vi "Convert to GRobot.vi"(8 "error in (no error)":errorcluster, 10 "scale":dbl=1.0, 11 "Robot In":refnum<class "NI_Robotics_Serial Robot Arm.lvclass">) -> (0 "error out":errorcluster, 2 "Robot Elements":T1[](array[typedef]), 3 "Robot Out":refnum<class "NI_Robotics_Serial Robot Arm.lvclass">)   [LabVIEW 2017, in "NI_Robotics_3DKinematics.lvlib"]
uses:
  <vilib>/robotics/Kinematics/Plotting/NI_Robotics_3DKinematics.lvlib
  <vilib>/robotics/Kinematics/Plotting/Tree Element.ctl
  <vilib>/robotics/Kinematics/Plotting/Element Type.ctl
  <vilib>/robotics/Kinematics/Plotting/Joint Type.ctl
  <vilib>/robotics/Kinematics/Robot/NI_Robotics_Serial Robot Arm.lvclass
  <vilib>/robotics/Kinematics/Link/Joint Type.ctl
  <vilib>/robotics/Kinematics/DH Convention.ctl
  <vilib>/Analysis/baseanly.llb/A x Vector.vi
  <vilib>/Analysis/_algsub.llb/Real Vector Norm.vi
  <vilib>/Utility/AngleManip/Radians to Degrees (Scalar DBL).vi
  <vilib>/robotics/Kinematics/NI_Kinematics.lvlib
  <vilib>/robotics/Kinematics/Link/NI_Robotics_Link.lvclass
  <vilib>/Analysis/NI_AALBase.lvlib
  <vilib>/Analysis/NI_AALPro.lvlib
  <vilib>/Utility/AngleManip/NI_AngleManipulation.lvlib
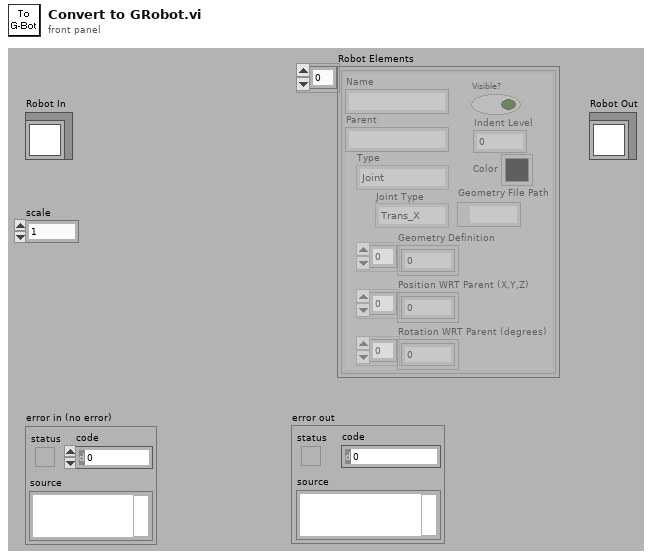
[diagram p1: front panel]
types:
  T1 = typedef "NI_Robotics_3DKinematics.lvlib/Tree Element.ctl" = cluster{"Name":string, "Parent":string, "Type":T2, "Visible?":bool, "Geometry Definition":dbl[], "Position WRT Parent (X,Y,Z)":dbl[], "Rotation WRT Parent (degrees)":dbl[], "Joint Type":T3, "Geometry File Path":path, "Indent Level":i32, "Color":u32}
  T2 = typedef "NI_Robotics_3DKinematics.lvlib/Element Type.ctl" = enum16{"Joint", "Box", "Cylinder", "Cone", "Sphere", "ASE File", "VRML File", "STL File", "Space"}
  T3 = typedef "NI_Robotics_3DKinematics.lvlib/Joint Type.ctl" = enum16{"Trans_X", "Trans_Y", "Trans_Z", "Rot_X", "Rot_Y", "Rot_Z", "None"}
  T4 = typedef "NI_Matrix.lvlib/RealMatrix.ctl" = dbl[][]
  T5 = typedef "NI_Robotics_Link.lvclass/Joint Type.ctl" = enum16{"Revolute", "Prismatic"}
  T6 = typedef "NI_Kinematics.lvlib/DH Convention.ctl" = enum16{"Standard", "Modified"}
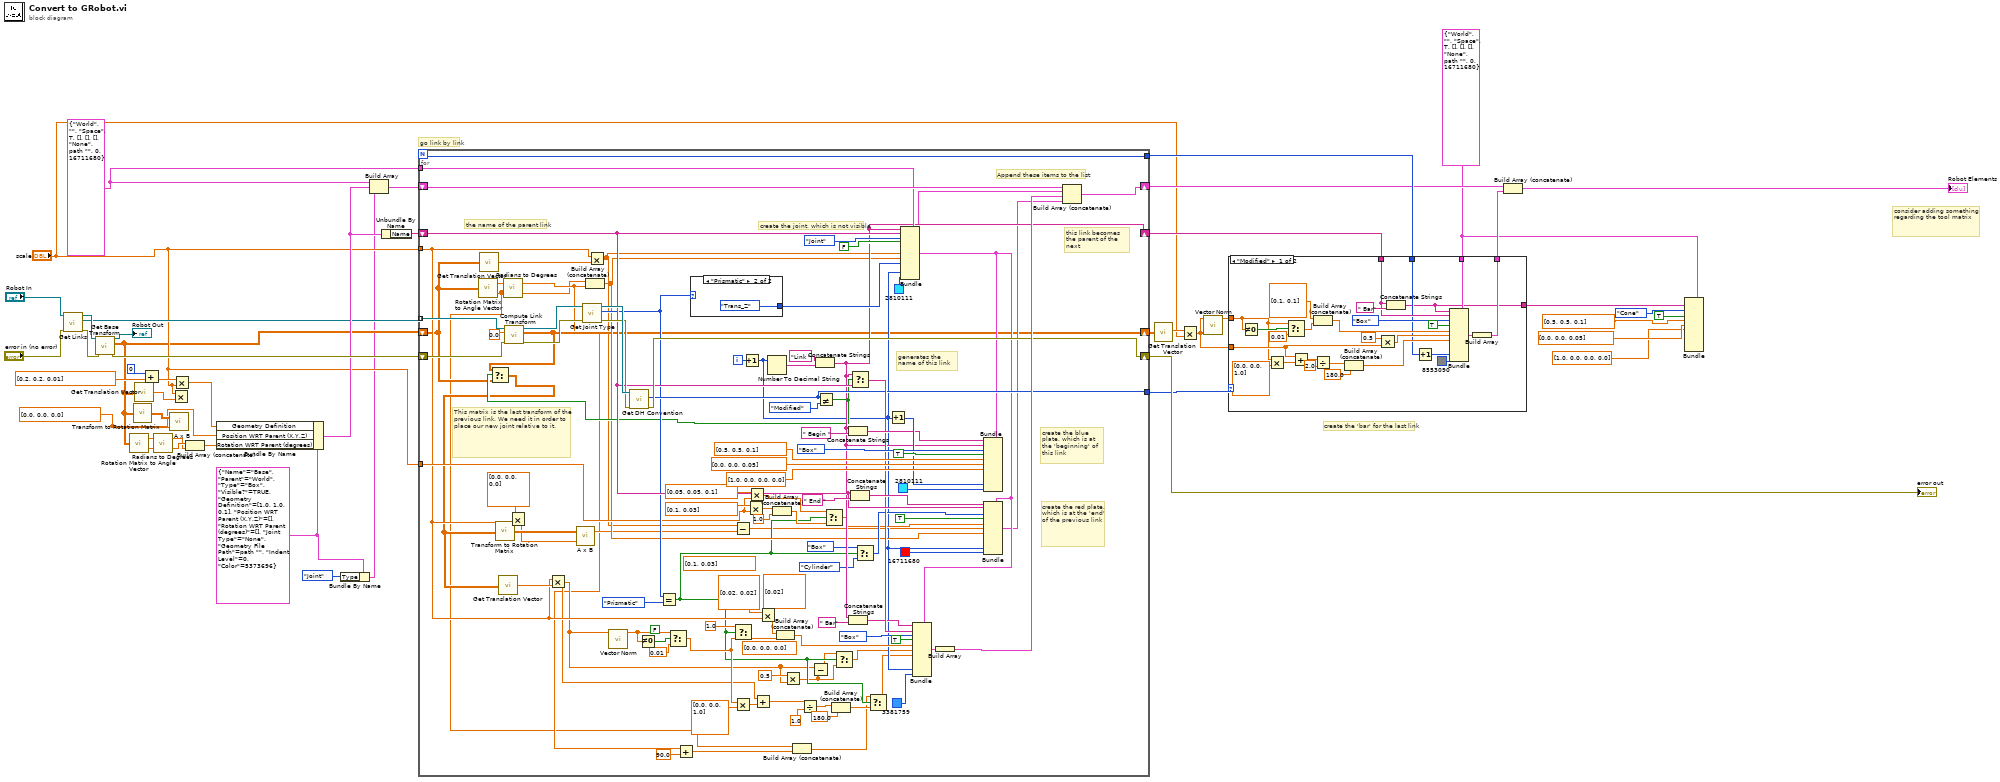
[diagram p0: block diagram]
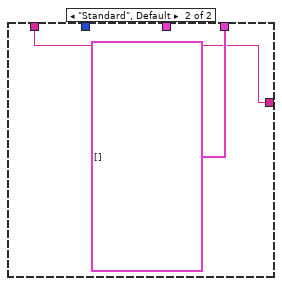
[diagram p2: hidden frame]
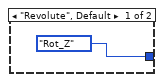
[diagram p3: hidden frame]
diagram:
  w5 = dbl[] [0.0, 0.0, 0.0] ("Geometry Definition")
  w4 = T1 {"Name"="Base", "Parent"="World", "Type"=enum."Box", "Visible?"=TRUE, "Geometry Definition"=[1.0, 1.0, 0.1], "Position WRT Parent (X,Y,Z)"=[], "Rotation WRT Parent (degrees)"=[], "Joint Type"=enum."None", "Geometry File Path"=path "", "Indent Level"=0, "Color"=5373696} ("Robot Element 2")
  w24 = T1 {"Name"="World", "Parent"="", "Type"=enum."Space", "Visible?"=TRUE, "Geometry Definition"=[], "Position WRT Parent (X,Y,Z)"=[], "Rotation WRT Parent (degrees)"=[], "Joint Type"=enum."None", "Geometry File Path"=path "", "Indent Level"=0, "Color"=16711680} ("Robot Element 2")
  w35 = T1 {"Name"="World", "Parent"="", "Type"=enum."Space", "Visible?"=TRUE, "Geometry Definition"=[], "Position WRT Parent (X,Y,Z)"=[], "Rotation WRT Parent (degrees)"=[], "Joint Type"=enum."None", "Geometry File Path"=path "", "Indent Level"=0, "Color"=16711680} ("Robot Element 2")
  # "consider adding something regarding the tool matrix"
  # "create the 'bar' for the last link"
  # "go link by link"
  n1 = call <vilib>:"Get Links.vi"("error in (no error)"="error in (no error)", "serial arm in"="Robot In") -> ("error out"=w32:errorcluster, "links"=w8:refnum<class "NI_Robotics_Link.lvclass">[], "serial arm out"=w31:refnum<class "NI_Robotics_Serial Robot Arm.lvclass">)  [unwired: 7 in]
  n2 = call <vilib>:"Get Base Transform.vi"("error in (no error)"=w32, "serial arm in"=w31) -> ("error out"=w29:errorcluster, "base transform"=w6:T4, "serial arm out"=→"Robot Out":refnum<class "NI_Robotics_Serial Robot Arm.lvclass">)  [unwired: 7 in]
  n3 = call <vilib>:"Rotation Matrix to Angle Vector.vi"("rotation matrix"=w6) -> ("angle"=w20:dbl, "vector"=w27:dbl[])
  n4 = call <vilib>:"Transform to Rotation Matrix.vi"("transform"=w6) -> ("rotation matrix"=w25:T4)
  n5 = call <vilib>:"Get Translation Vector.vi"("transform"=w6) -> ("translation vector"=w9:dbl[])
  n6 = Add(x=0 ("Numeric"), y=dbl[] [0.2, 0.2, 0.01] ("Geometry Definition")) -> (x+y=w11:dbl[])
  n7 = call-poly <vilib>:"Radians to Degrees.vi"("angle (rad)"=w20) -> ("angle (deg)"=w19:dbl)  [unwired: 2 in]
  n8 = call-poly <vilib>:"A x B.vi"("Vector"=w5, "A"=w25) -> ()  [unwired: 2 out]
  n9 = Multiply(x="scale", y=w9) -> ()  [unwired: 1 out]
  n10 = Multiply(x=w11, y="scale") -> (x*y=w12:dbl[])
  n11 = Build Array (concatenate)(w27, w19) -> (w26:dbl[])
  n12 = Bundle By Name(cluster=w4, "Geometry Definition"=w12, "Position WRT Parent (X,Y,Z)"=w5, "Rotation WRT Parent (degrees)"=w26) -> (w17:T1)
  n13 = Bundle By Name(cluster=w4, "Type"=Element_Type."Joint") -> (w2:T1)
  n14 = Build Array(w35, w17, w2) -> (w45:T1[])
  n15 = Unbundle By Name(w17) -> ("Name"=w34:string)
  n16 = for {
    N -> [w77]
    tunnel: w8 -> [w127] mode=indexing
    shift-right: [w145] -> w41
    shift-left: w45 -> [w146]
    tunnel: w35 -> [w144]
    shift-right: [w107] -> w42
    shift-left: w34 -> [w113]
    shift-right: [w74] -> w44
    shift-left: w6 -> [w56]
    tunnel: [w77] -> w43
    tunnel: "scale" -> [w78]
    shift-right: [w114] -> w28
    shift-left: w29 -> [w120]
    tunnel: [w110] -> w18
    tunnel: "scale" -> [w84]
    i -> [w76]
    (unwired) dbl[] [0.02] ("Geometry Definition")
    (unwired) FALSE ("s")
    (unwired) dbl[] [0.1, 0.03] ("Geometry Definition")
    (unwired) dbl[] [0.0, 0.0, 0.0] ("t")
    # "create the joint, which is not visible"
    # "this link becomes the parent of the next"
    # "generates the name of this link"
    # "create the red plate, which is at the 'end' of the previous link"
    # "create the blue plate, which is at the 'beginning' of this link"
    # "Append these items to the list"
    # "the name of the parent link"
    # "This matrix is the last transform of the previous link. We need it in order to place our new joint relative to it."
    n17 = call <vilib>:"Rotation Matrix to Angle Vector.vi"("rotation matrix"=w56) -> ("angle"=w117:dbl, "vector"=w47:dbl[])
    n18 = call <vilib>:"Get Translation Vector.vi"("transform"=w56) -> ("translation vector"=w121:dbl[])
    n19 = call-poly <vilib>:"Radians to Degrees.vi"("angle (rad)"=w117) -> ("angle (deg)"=w48:dbl)  [unwired: 2 in]
    n20 = call <vilib>:"Compute Link Transform.vi"("error in (no error)"=w120, "q"=0.0, "Link in"=w127) -> ("error out"=w119:errorcluster, "Link Transform"=w74:T4, "Link out"=w118:refnum<class "NI_Robotics_Link.lvclass">)  [unwired: 6 in]
    n21 = Multiply(x=dbl[] [0.0, 0.0, 0.0] ("Geometry Definition"), y=w78) -> (x*y=w91:dbl[])
    n22 = call <vilib>:"Get Joint Type.vi"("error in (no error)"=w119, "Link in"=w118) -> ("error out"=w115:errorcluster, "Joint Type"=w108:T5, "Link out"=w116:refnum<class "NI_Robotics_Link.lvclass">)  [unwired: 7 in]
    n23 = Build Array (concatenate)(w47, w48) -> (w80:dbl[])
    n24 = Multiply(x=w78, y=w121) -> (x*y=w52:dbl[])
    n25 = call <vilib>:"Get DH Convention.vi"("error in (no error)"=w115, "Link In"=w116) -> ("error out"=w114:errorcluster, "DH Convention"=w110:T6)  [unwired: 7 in, 1 out]
    n26 = Equal?(x=w108, y=Joint_Type."Prismatic" ("Joint Type")) -> (x = y?=w63:bool)
    n27 = Add(x=w48, y=90.0) -> (x+y=w54:dbl)
    n28 = case shown="\"Prismatic\"" w108 {
      tunnel: [Joint_Type."Rot_Z" ("Joint Type") Joint_Type."Trans_Z" ("Joint Type")] -> w141
      frame "Revolute", Default {
      }
      frame "Prismatic" {
      }
    }
    n29 = Increment(x=w76) -> (x+1=w75:i32)
    n30 = Multiply(x=dbl[] [0.1, 0.03] ("Geometry Definition"), y=w84) -> (x*y=w93:dbl[])
    n31 = Multiply(x=dbl[] [0.05, 0.05, 0.1] ("Geometry Definition"), y=w84) -> (x*y=w81:dbl[])
    n32 = Multiply(x=dbl[] [0.02, 0.02] ("Geometry Definition"), y=w78) -> (x*y=w90:dbl[])
    n33 = Number To Decimal String(number=w75) -> (decimal integer string=w147:string)  [unwired: 1 in]
    n34 = Build Array (concatenate)(w93, 1.0 ("Numeric")) -> (w86:dbl[])
    n35 = Build Array (concatenate)(w47, w54) -> (w55:dbl[])
    n36 = Concatenate Strings("Link ", w147) -> (w107:string)
    n37 = Not Equal?(x=w110, y=DH_Convention."Modified" ("DH Convention")) -> (x != y?=w82:bool)
    n38 = Select(t=w74, s=w82, f=w56) -> (s? t:f=w61:T4)
    n39 = call <vilib>:"Transform to Rotation Matrix.vi"("transform"=w61) -> ("rotation matrix"=w123:T4)
    n40 = call <vilib>:"Get Translation Vector.vi"("transform"=w61) -> ("translation vector"=w79:dbl[])
    n41 = Multiply(x=w78, y=w79) -> (x*y=w49:dbl[])
    n42 = call-poly <vilib>:"A x B.vi"("Vector"=w91, "A"=w123) -> ("A x Vector"=w73:dbl[])  [unwired: 1 out]
    n43 = call-poly <vilib>:"Vector Norm.vi"("Input Vector"=w49) -> ("norm"=w96:dbl)  [unwired: 9 in, 1 out]
    n44 = Not Equal To 0?(x=w96) -> (x != 0?=w72:bool)
    n45 = Select(t=w96, s=w72, f=0.01) -> (s? t:f=w65:dbl)
    n46 = Multiply(x=w65, y=dbl[] [0.0, 0.0, 1.0] ("Geometry Definition")) -> (x*y=w59:dbl[])
    n47 = Subtract(x=w52, y=w73) -> (x-y=w50:dbl[])
    n48 = Select(t=1.0 ("f"), s=w63, f=w65) -> (s? t:f=w97:dbl)
    n49 = Add(x=w49, y=w59) -> (x+y=w60:dbl[])
    n50 = Build Array (concatenate)(w90, w97) -> (w101:dbl[])
    n51 = Multiply(x=0.5 ("f"), y=w49) -> (x*y=w46:dbl[])
    n52 = Divide(x=w60, y=1.0) -> (x/y=w67:dbl[])
    n53 = Subtract(x=w49, y=w46) -> (x-y=w51:dbl[])
    n54 = Select(t=w81, s=w63, f=w86) -> (s? t:f=w85:dbl[])
    n55 = Build Array (concatenate)(w67, 180.0) -> (w57:dbl[])
    n56 = Select(t=w51, s=w63, f=w46) -> (s? t:f=w70:dbl[])
    n57 = Concatenate Strings(w107, " Begin ") -> (w129:string)
    n58 = Concatenate Strings(w107, " Bar" ("string")) -> (w106:string)
    n59 = Select(t=w107, s=w82, f=w113) -> (s? t:f=w112:string)
    n60 = Concatenate Strings(w113, " End ") -> (w128:string)
    n61 = Select(t=Element_Type."Box" ("Type"), s=w63, f=Element_Type."Cylinder" ("Type")) -> (s? t:f=w88:T2)
    n62 = Select(t=w55, s=w63, f=w57) -> (s? t:f=w62:dbl[])
    n63 = Increment(x=w75) -> (x+1=w131:i32)
    n64 = Bundle(cluster=w144, "Name"=w107, "Parent"=w113, "Type"=Element_Type."Joint", "Visible?"=FALSE ("Visable?"), "Position WRT Parent (X,Y,Z)"=w52, "Rotation WRT Parent (degrees)"=w80, "Joint Type"=w141, "Indent Level"=w75, "Color"=u32 2810111) -> (w95:T1)  [unwired: 2 in]
    n65 = Bundle(cluster=w95, "Name"=w106, "Parent"=w112, "Type"=Element_Type."Box", "Visible?"=TRUE ("Visable?"), "Geometry Definition"=w101, "Position WRT Parent (X,Y,Z)"=w70, "Rotation WRT Parent (degrees)"=w62, "Indent Level"=w75, "Color"=u32 3381759) -> (w98:T1)  [unwired: 2 in]
    n66 = Build Array(w98) -> (w122:T1[])
    n67 = Bundle(cluster=w95, "Name"=w129, "Parent"=w107, "Type"=Element_Type."Box", "Visible?"=TRUE ("Visable?"), "Geometry Definition"=dbl[] [0.5, 0.5, 0.1], "Position WRT Parent (X,Y,Z)"=dbl[] [0.0, 0.0, 0.05], "Rotation WRT Parent (degrees)"=dbl[] [1.0, 0.0, 0.0, 0.0] ("Position WRT Parent (X,Y,Z)"), "Indent Level"=w131, "Color"=u32 2810111) -> ()  [unwired: 2 in, 1 out]
    n68 = Bundle(cluster=w95, "Name"=w128, "Parent"=w113, "Type"=w88, "Visible?"=TRUE ("Visable?"), "Geometry Definition"=w85, "Position WRT Parent (X,Y,Z)"=w50, "Rotation WRT Parent (degrees)"=w80, "Indent Level"=w75, "Color"=u32 16711680) -> (w94:T1)  [unwired: 2 in]
    n69 = Build Array (concatenate)(w146, w95, w122, w94) -> (w145:T1[])
  }
  "error out" <- w28
  n70 = call <vilib>:"Get Translation Vector.vi"("transform"=w44) -> ("translation vector"=w37:dbl[])
  n71 = Multiply(x=w37, y="scale") -> (x*y=w36:dbl[])
  n72 = call-poly <vilib>:"Vector Norm.vi"("Input Vector"=w36) -> ("norm"=w38:dbl)  [unwired: 9 in, 1 out]
  n73 = case shown="\"Modified\"" w18 {
    tunnel: w38 -> [w151 _]
    tunnel: w36 -> [w162 _]
    tunnel: w24 -> [w161 _]
    tunnel: w43 -> [w156 _]
    tunnel: w42 -> [w160 w178]
    tunnel: [w158 T1[] []] -> w39
    tunnel: [w155 w178] -> w23
    frame "Modified" {
      n74 = Not Equal To 0?(x=w151) -> (x != 0?=w154:bool)
      n75 = Multiply(x=w151, y=dbl[] [0.0, 0.0, 1.0] ("Geometry Definition")) -> (x*y=w173:dbl[])
      n76 = Select(t=w151, s=w154, f=0.01) -> (s? t:f=w152:dbl)
      n77 = Add(x=w162, y=w173) -> (x+y=w172:dbl[])
      n78 = Build Array (concatenate)(dbl[] [0.1, 0.1] ("Geometry Definition"), w152) -> (w169:dbl[])
      n79 = Divide(x=w172, y=2.0) -> (x/y=w166:dbl[])
      n80 = Build Array (concatenate)(w166, 180.0) -> (w167:dbl[])
      n81 = Multiply(x=0.5, y=w162) -> (x*y=w168:dbl[])
      n82 = Concatenate Strings(w160, " Bar" ("string")) -> (w155:string)
      n83 = Increment(x=w156) -> (x+1=w157:i32)
      n84 = Bundle(cluster=w161, "Name"=w155, "Parent"=w160, "Type"=Element_Type."Box", "Visible?"=TRUE ("Visable?"), "Geometry Definition"=w169, "Position WRT Parent (X,Y,Z)"=w168, "Rotation WRT Parent (degrees)"=w167, "Indent Level"=w157, "Color"=u32 8553090) -> (w159:T1)  [unwired: 2 in]
      n85 = Build Array(w159) -> (w158:T1[])
    }
    frame "Standard", Default {
    }
  }
  n86 = Build Array (concatenate)(w41, w39) -> (→"Robot Elements":T1[])
  n87 = Bundle(cluster=w24, "Parent"=w23, "Type"=Element_Type."Cone", "Visible?"=TRUE ("Visable?"), "Geometry Definition"=dbl[] [0.5, 0.5, 0.1], "Position WRT Parent (X,Y,Z)"=dbl[] [0.0, 0.0, 0.05], "Rotation WRT Parent (degrees)"=dbl[] [1.0, 0.0, 0.0, 0.0] ("Position WRT Parent (X,Y,Z)")) -> ()  [unwired: 5 in, 1 out]
